vi "Write Name.vi"(10 "Name":string, 11 "((Pointer)) in":refnum<class "_Pointer.lvclass">) -> (3 "((Pointer)) out":refnum<class "_Pointer.lvclass">)   [LabVIEW 2020, in "_Pointer.lvclass"]
uses:
  _Pointer.lvclass
  _Pointer.lvclass/_Pointer.ctl
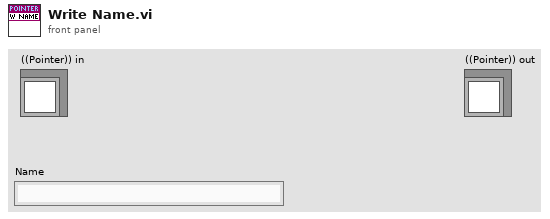
[diagram p1: front panel]
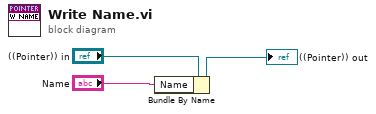
[diagram p0: block diagram]
diagram:
  n1 = Bundle By Name(cluster="((Pointer)) in", "Name"="Name") -> (→"((Pointer)) out":refnum<class "_Pointer.lvclass">)
